vi "normalise.vi"(1 "amplitude matrix":cdb[][](array[numeric]) format="%.2f") -> (0 "normalised amplitude matrix":cdb[][](array[numeric]) format="%.2f")   [LabVIEW 2024]
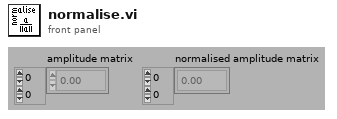
[diagram p1: front panel]
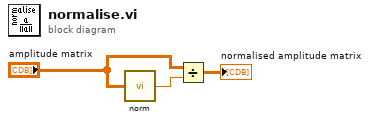
[diagram p0: block diagram]
diagram:
  n1 = call "norm.vi"("amplitude matrix"="amplitude matrix") -> ("norm"=w3:dbl)
  n2 = Divide(x="amplitude matrix", y=w3) -> (x/y=→"normalised amplitude matrix":cdb[][])
